vi "GlobalCameraHandle.vi"() -> ()   [LabVIEW 2009]
panel:
  in  "CameraHandle":dbl
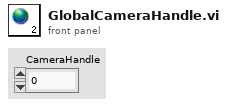
[diagram p1: front panel]
diagram:
